vi "conv temp.vi"() -> ()   [LabVIEW 2015]
panel:
  in  "input":i16=2048
  out "output":dbl format="%#_6f"
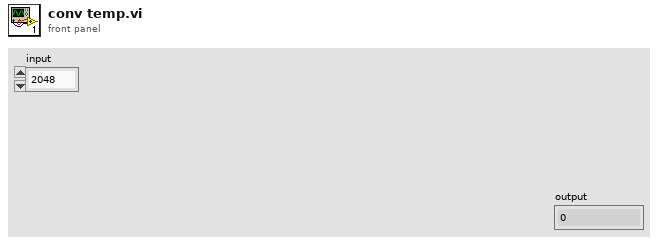
[diagram p1: front panel]
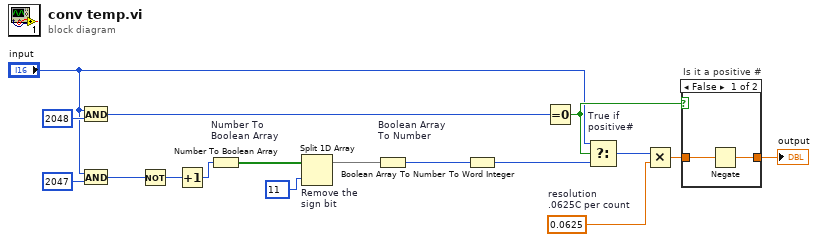
[diagram p0: block diagram]
diagram:
  w17 = 0.0625  # resolution .0625C per count
  n1 = And ("Out = 0x800\nif neg #")(x="input", y=u16 2048 ("number 2")) -> (x .and. y?=w14:u16)
  n2 = And ("Just the \n12 bits")(x="input", y=i16 2047 ("number")) -> (x .and. y?=w3:i16)
  n3 = Not(x=w3) -> (.not. x?=w13:i16)
  n4 = Increment(x=w13) -> (x+1=w12:i16)
  n5 = Number To Boolean Array "Number To\nBoolean Array"(number=w12) -> (Boolean array=w11:bool[])
  n6 = Split 1D Array "Remove the \nsign bit"(array=w11, index=11) -> (first subarray=w4:bool[])  [unwired: 1 out]
  n7 = Boolean Array To Number "Boolean Array \nTo Number"(Boolean array=w4) -> (number=w9:u32)
  n8 = To Word Integer(number=w9) -> (16bit integer=w8:i16)
  n9 = Equal To 0?(x=w14) -> (x = 0?=w7:bool)
  n10 = Select "True if \npositive#"(t="input", s=w7, f=w8) -> (s? t:f=w15:i16)
  n11 = Multiply(x=w15, y=w17) -> (x*y=w6:dbl)
  n12 = case "Is it a positive #" shown="False" w7 {
    tunnel: w6 -> [w19 w20]
    tunnel: [w18 w20] -> w5
    frame False {
      n13 = Negate(x=w19) -> (-x=w18:dbl)
    }
    frame True {
    }
  }
  "output" <- w5
